vi "Find Delta Samples of Rising Edge.vi"(10 "Channel 2":waveform(dbl), 11 "Channel 1":waveform(dbl)) -> (3 "Sample Offset":dbl)   [LabVIEW 2025]
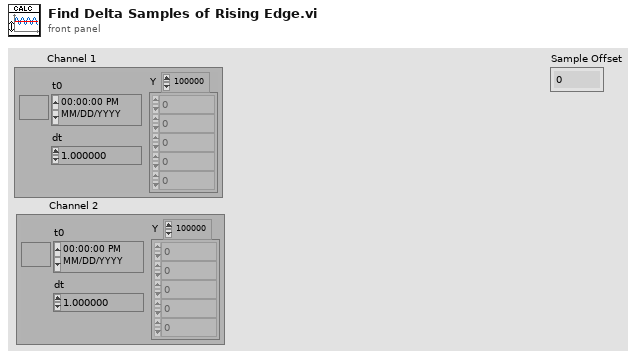
[diagram p1: front panel]
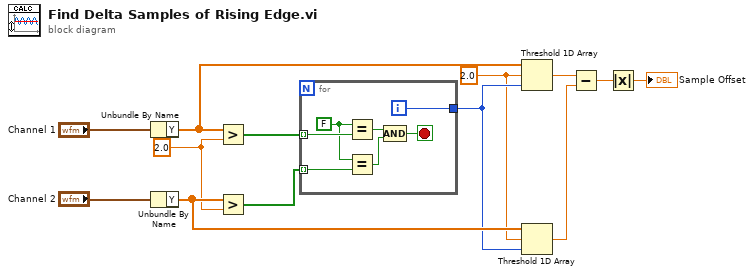
[diagram p0: block diagram]
diagram:
  w2 = 2.0 ("threshold y")
  w3 = 2.0
  n1 = Unbundle By Name("Channel 1") -> ("Y"=w11:dbl[])
  n2 = Unbundle By Name("Channel 2") -> ("Y"=w10:dbl[])
  n3 = Greater?(x=w11, y=w3) -> (0:w6:bool[])
  n4 = Greater?(x=w10, y=w3) -> (0:w5:bool[])
  n5 = for {
    tunnel: w6 -> [w20] mode=indexing
    tunnel: w5 -> [w19] mode=indexing
    tunnel: [w18] -> w4
    i -> [w18]
    stop <- w15 stop-if-true
    w14 = FALSE ("x")
    n6 = Equal?(x=w14, y=w20) -> (x = y?=w17:bool)
    n7 = Equal?(x=w14, y=w19) -> (x = y?=w16:bool)
    n8 = Compound Arithmetic op=AND(w17, w16) -> (w15:bool)
  }
  n9 = Threshold 1D Array(1:w4, 2:w2, 3:w11) -> (0:w9:dbl)
  n10 = Threshold 1D Array(1:w4, 2:w2, 3:w10) -> (0:w8:dbl)
  n11 = Subtract(x=w9, y=w8) -> (x-y=w7:dbl)
  n12 = Absolute Value(x=w7) -> (abs(x)=→"Sample Offset":dbl)
